vi "Create Buffers.vi"(7 "framework configuration":T1, 8 "error in (no error)":errorcluster, 11 "Framework in":refnum<class "Framework.lvclass">) -> (0 "error out":errorcluster, 3 "Framework out":refnum<class "Framework.lvclass">)   [LabVIEW 2017, in "DSF Core.lvlib" / "Framework.lvclass"]
uses:
  Framework.lvclass
  DSF Configuration API/Public/Controls/DSF Engine Framework Configuration.ctl
  DSF Configuration API/Public/Controls/DSF Engine Plugin Configuration.ctl
  DSF Configuration API/Public/Controls/DSF Timing Info.ctl
  DSF Configuration API/Public/Controls/DSF Engine Transfer Group Configuration.ctl
  DSF Configuration API/Public/Controls/DSF Direction.ctl
  DSF Configuration API/Public/Controls/DSF Engine Transfer Configuration.ctl
  DSF Configuration API/Public/Controls/DSF Byte Order.ctl
  DSF Configuration API/Public/Controls/DSF Engine Channel Configuration.ctl
  DSF Configuration API/Public/Controls/DSF Data Type.ctl
  DSF Configuration API/Public/Controls/DSF Settings Info.ctl
  Framework.lvclass/Framework.ctl
  Shared/VIs/Sizeof.vi
  DSF Configuration API/Public/Required Buffer Size (Framework).vi
  DSF Configuration API/Public/Channel Count (Framework).vi
  Buffer/Buffer.lvclass
  Buffer/Buffers.lvclass
  DSF Core.lvlib
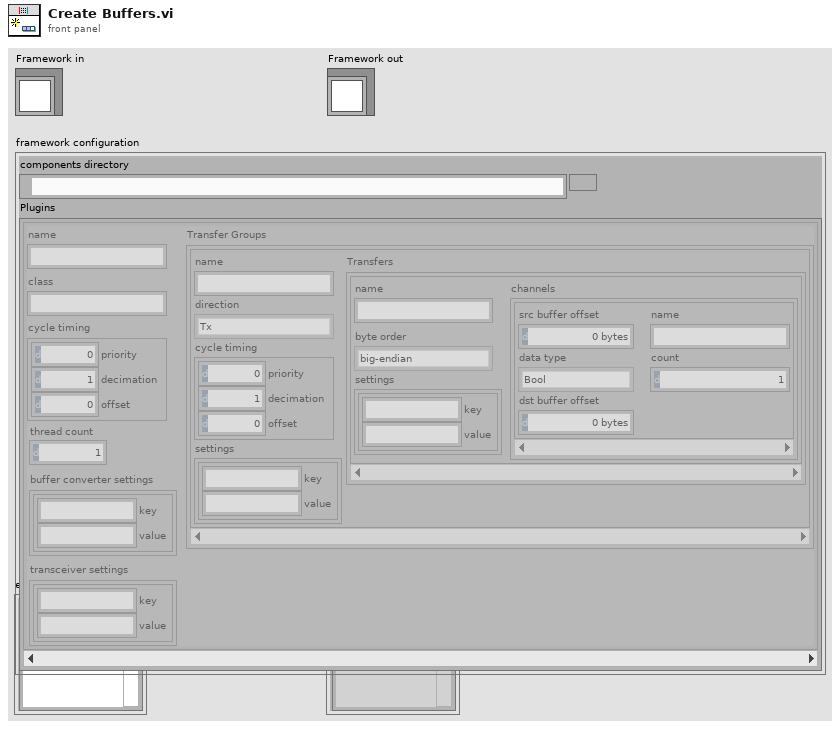
[diagram p1: front panel]
types:
  T1 = typedef "DSF Core.lvlib/DSF Engine Framework Configuration.ctl" = cluster{"components directory":path, "Plugins":T2[]}
  T2 = typedef "DSF Core.lvlib/DSF Engine Plugin Configuration.ctl" = cluster{"name":string, "class":string, "cycle timing":T3, "Transfer Groups":T4[], "thread count":i32, "buffer converter settings":T10, "transceiver settings":T10}
  T3 = typedef "DSF Core.lvlib/DSF Timing Info.ctl" = cluster{"priority":u64, "decimation":u64, "offset":u64}
  T4 = typedef "DSF Core.lvlib/DSF Engine Transfer Group Configuration.ctl" = cluster{"name":string, "direction":T5, "cycle timing":T3, "Transfers":T6[], "settings":T10}
  T5 = typedef "DSF Core.lvlib/DSF Direction.ctl" = enum8{"Tx", "Rx"}
  T6 = typedef "DSF Core.lvlib/DSF Engine Transfer Configuration.ctl" = cluster{"name":string, "byte order":T7, "channels":T8[], "settings":T10}
  T7 = typedef "DSF Core.lvlib/DSF Byte Order.ctl" = enum8{"big-endian", "little-endian"}
  T8 = typedef "DSF Core.lvlib/DSF Engine Channel Configuration.ctl" = cluster{"src buffer offset":u64, "name":string, "data type":T9, "count":u64, "dst buffer offset":u64}
  T9 = typedef "DSF Core.lvlib/DSF Data Type.ctl" = enum8{"Bool", "SGL", "DBL", "I8", "I16", "I32", "I64", "U8", "U16", "U32", "U64"}
  T10 = typedef "DSF Core.lvlib/DSF Settings Info.ctl" = cluster{"key":string, "value":string}[]
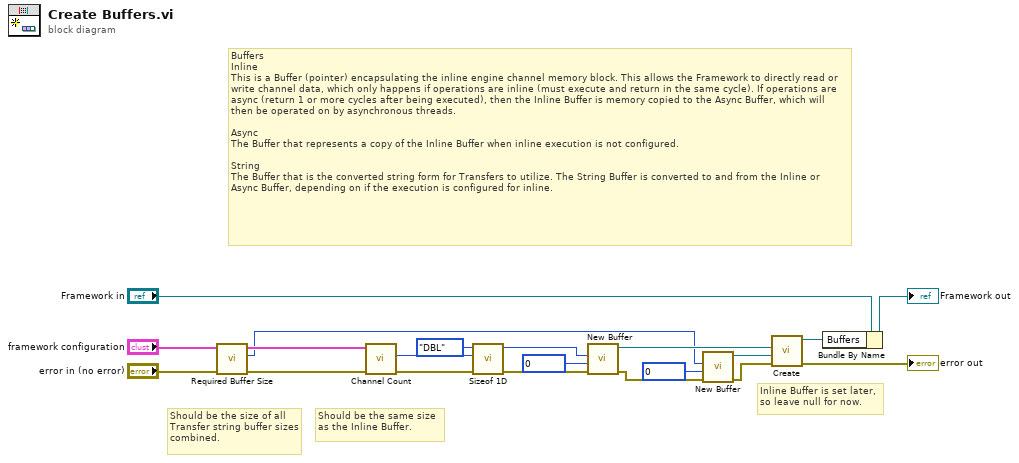
[diagram p0: block diagram]
diagram:
  # "Should be the size of all Transfer string buffer sizes combined."
  # "Should be the same size as the Inline Buffer."
  # "Buffers\nInline\nThis is a Buffer (pointer) encapsulating the inline engine channel memory block. This allows the Framework to directly read or write channel data, which only happens if operations are inline (must execute and return in the same cycle). If operations are async (return 1 or more cycles after being executed), then the Inline Buffer is memory copied to the Async Buffer, which will then be operated on by asynchronous threads.\n\nAsync\nThe Buffer that represents a copy of the Inline Buffer when inline execution is not configured.\n\nString\nThe Buffer that is the converted string form for Transfers to utilize. The String Buffer is converted to and from the Inline or Async Buffer, depending on if the execution is configured for inline."
  # "Inline Buffer is set later, so leave null for now."
  n1 = call-poly "Required Buffer Size.vi"("error in (no error)"="error in (no error)", "Framework Configuration in"="framework configuration") -> ("error out"=w12:errorcluster, "required buffer size"=w5:u64, "Framework Configuration out"=w13:T1)  [unwired: 7 in]
  n2 = call-poly "Channel Count.vi"("error in (no error)"=w12, "Framework Configuration in"=w13) -> ("error out"=w1:errorcluster, "total channel count"=w4:u64)  [unwired: 7 in, 1 out]
  n3 = call "Sizeof 1D.vi"("count"=w4, "data type"=DSF_Data_Type."DBL") -> ("size in bytes"=w2:u64)  [unwired: 9 in]
  n4 = call "New Buffer.vi"("error in (no error)"=w1, "buffer offset"=u64 0, "buffer size"=w2) -> ("error out"=w16:errorcluster, "Buffer out"=w7:refnum<class "Buffer.lvclass">)  [unwired: 7 in]
  n5 = call "New Buffer.vi"("error in (no error)"=w16, "buffer offset"=u64 0, "buffer size"=w5) -> ("error out"=w19:errorcluster, "Buffer out"=w15:refnum<class "Buffer.lvclass">)  [unwired: 7 in]
  n6 = call "Create.vi"("error in (no error)"=w19, "String Buffer (null)"=w15, "Async Buffer (null)"=w7) -> ("error out"=→"error out":errorcluster, "Buffers out"=w18:refnum<class "Buffers.lvclass">)  [unwired: 7 in]
  n7 = Bundle By Name(cluster="Framework in", "Buffers"=w18) -> (→"Framework out":refnum<class "Framework.lvclass">)
